vi "myRIO_BRig_RT_dataExp_SolenoidProbability_R.vi"() -> (2 "output_SolenoidProbability_R":i32)   [LabVIEW 2014]
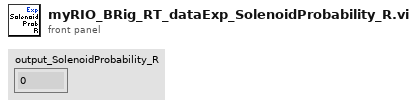
[diagram p1: front panel]
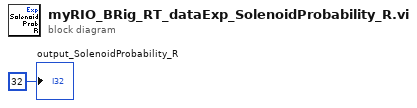
[diagram p0: block diagram]
diagram:
  "output_SolenoidProbability_R" <- 32 ("output_iBlock")
